vi "Handle IDN.vi"(8 "error in (no error)":errorcluster, 11 "Instrument in":refnum<class "Instrument.lvclass">) -> (0 "error out":errorcluster, 2 "IDN":T1, 3 "Instrument out":refnum<class "Instrument.lvclass">)   [LabVIEW 2019, in "Instrument.lvclass"]
uses:
  Instrument.lvclass
  Typedefs/Instrument.IDN--cluster.ctl
  Instrument.lvclass/Instrument.ctl
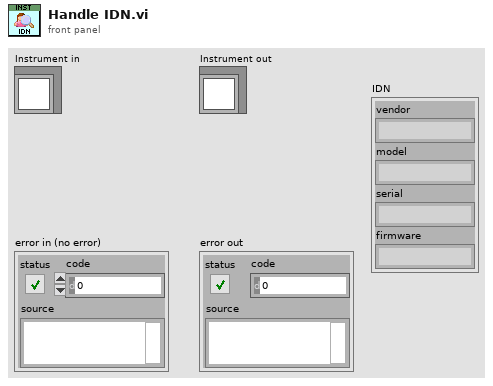
[diagram p1: front panel]
types:
  T1 = typedef "Instrument.lvclass/Instrument.IDN--cluster.ctl" = cluster{"vendor":string, "model":string, "serial":string, "firmware":string}
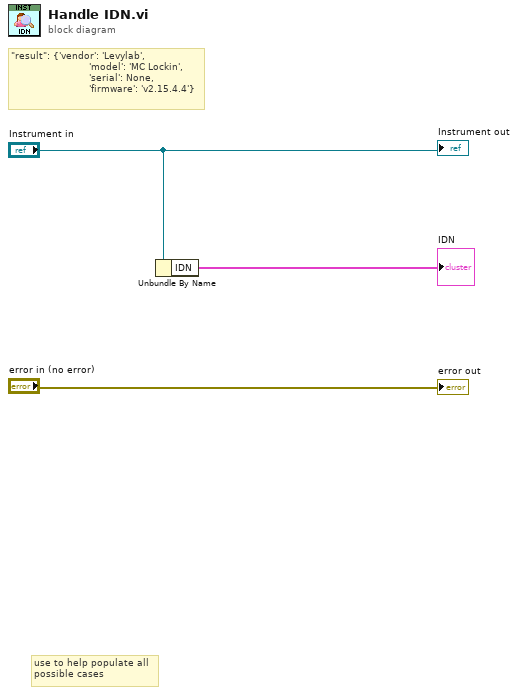
[diagram p0: block diagram]
diagram:
  # "\"result\": {'vendor': 'Levylab',\n                          'model': 'MC Lockin',\n                          'serial': None,\n                          'firmware': 'v2.15.4.4'}"
  # "use to help populate all\npossible cases"
  n1 = Unbundle By Name("Instrument in") -> ("IDN"=→"IDN":T1)
  "Instrument out" <- "Instrument in"
  "error out" <- "error in (no error)"
